vi "Query Status Byte.vi"(8 "error in (no error)":errorcluster, 10 "Query extended status? (F)":bool, 11 "VISA resource name":refnum<visa-resource-name>) -> (0 "error out":errorcluster, 2 "Status Register":T1, 3 "VISA resource name out":refnum<visa-resource-name>)   [LabVIEW 2015, in "SR400.lvlib"]
doc: "Query status byte."
uses:
  SR400.lvlib
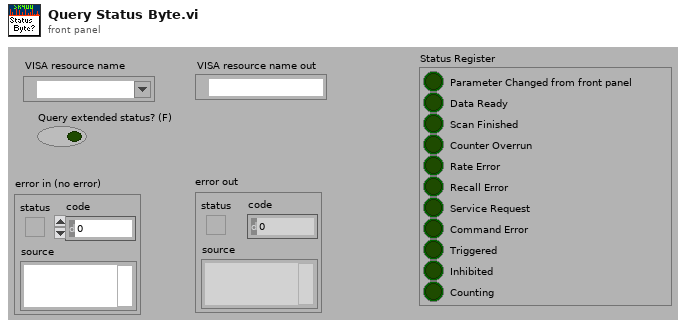
[diagram p1: front panel]
types:
  T1 = cluster{"Parameter Changed from front panel":bool, "Data Ready":bool, "Scan Finished":bool, "Counter Overrun":bool, "Rate Error":bool, "Recall Error":bool, "Service Request":bool, "Command Error":bool, "Triggered":bool, "Inhibited":bool, "Counting":bool}
  T2 = cluster{"[0]":bool, "[1]":bool, "[2]":bool, "[3]":bool, "[4]":bool, "[5]":bool, "[6]":bool, "[7]":bool, "[8]":bool, "[9]":bool, "[10]":bool}
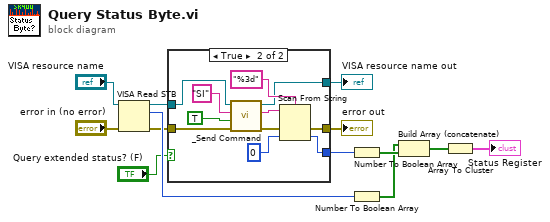
[diagram p0: block diagram]
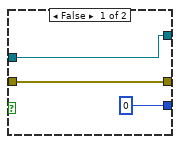
[diagram p2: hidden frame]
diagram:
  n1 = VISA Read STB(8:"error in (no error)", 11:"VISA resource name") -> (0:w3:errorcluster, 2:w4:u16, 3:w2:refnum<visa-resource-name>)
  n2 = case shown="True" "Query extended status? (F)" {
    tunnel: [w14 w20] -> w13
    tunnel: [w15 w26] -> w12
    tunnel: [u8 0 ("default value 1") w24] -> w11
    tunnel: w3 -> [w15 w21]
    tunnel: w2 -> [w14 w23]
    frame False {
    }
    frame True {
      n3 = call "_Send Command.vi"("error in (no error)"=w21, "Query? (F)"=TRUE, "Command"="SI" ("write buffer"), "VISA resource name"=w23) -> ("error out"=w18:errorcluster, "Response"=w19:string, "VISA resource name out"=w20:refnum<visa-resource-name>)  [unwired: 5 out]
      n4 = Scan From String(format string="%3d", input string=w19, error in=w18, default 1=u8 0 ("default value 1")) -> (error out=w26:errorcluster, output 1=w24:u8)  [unwired: 1 in, 2 out]
    }
  }
  "VISA resource name out" <- w13
  "error out" <- w12
  n5 = Number To Boolean Array(number=w11) -> (Boolean array=w10:bool[])
  n6 = Number To Boolean Array(number=w4) -> (Boolean array=w9:bool[])
  n7 = Build Array (concatenate)(w9, w10) -> (w8:bool[])
  n8 = Array To Cluster(array=w8) -> (cluster=→"Status Register":T2)
